vi "readcsv.vi"(0 "Order":i32=3, 1 "Baseline Data (optional)":path[](array[path])) -> (2 "B(x)":dbl[][](array[numeric]), 3 "Array":cluster{"all rows":dbl[], "all rows":dbl[]}[](array[cluster]), 4 "Names":string[](array[string]))   [LabVIEW 2013]
uses:
  <vilib>/Analysis/NI_AALPro.lvlib
  <vilib>/Utility/file.llb/Read Delimited Spreadsheet (DBL).vi
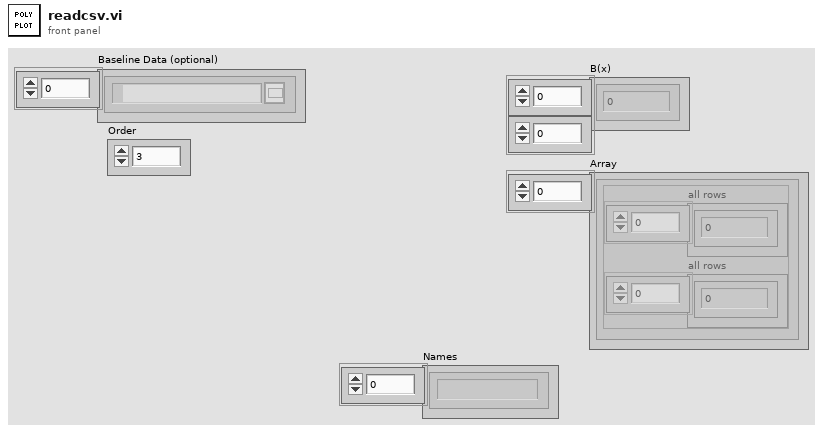
[diagram p1: front panel]
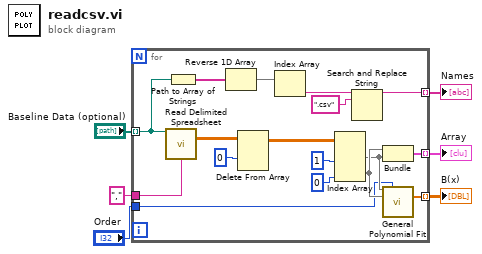
[diagram p0: block diagram]
diagram:
  n1 = for {
    tunnel: "," ("delimiter (\\t)") -> [w21]
    tunnel: "Baseline Data (optional)" -> [w15] mode=indexing
    tunnel: [w18] -> w4 mode=indexing
    tunnel: [w17] -> w3 mode=indexing
    tunnel: "Order" -> [w16]
    tunnel: [w10] -> w1 mode=indexing
    n2 = call-poly <vilib>:"Read Delimited Spreadsheet.vi"("file path (dialog if empty)"=w15, "delimiter (\\t)"=w21) -> ("all rows"=w9:dbl[][])  [unwired: 8 in, 5 out]
    n3 = Path to Array of Strings(0:w15) -> (2:w14:string[])  [unwired: 1 out]
    n4 = Reverse 1D Array(array=w14) -> (reversed array=w13:string[])
    n5 = Delete From Array(array=w9, index (row)=0) -> (array with subset deleted=w7:dbl[][])  [unwired: 2 in, 1 out]
    n6 = Index Array(array=w13) -> (element=w12:string)  [unwired: 1 in]
    n7 = Index Array(array=w7, index (col) #1=1 ("disabled index (col)"), index (col) #2=0 ("index (col)")) -> (element #1=w19:dbl[], element #2=w20:dbl[])  [unwired: 2 in]
    n8 = Search and Replace String(input string=w12, search string=".csv") -> (result string=w10:string)  [unwired: 6 in, 3 out]
    n9 = Bundle("all rows"=w20, "all rows"=w19) -> (w17:cluster{"all rows":dbl[], "all rows":dbl[]})  [unwired: 1 in]
    n10 = call <vilib>:"General Polynomial Fit.vi"("Y"=w19, "polynomial order"=w16, "X"=w20) -> ("Polynomial Coefficients"=w18:dbl[])  [unwired: 9 in, 3 out]
  }
  "B(x)" <- w4
  "Array" <- w3
  "Names" <- w1
